vi "Tokenize Json String.vi"(0 "JSON String":string="{\n   \"data\":[\n      {\n         \"message\":{\n            \"content\":{\n               \"type\":\"text/plain\",\n               \"text\":\"Some text asd\"\n            },\n            \"subject\":\"My subject\",\n            \"status\":\"published\",\n            \"replyCount\":4.8,\n            \"likeCount\":0.7\n         }\n      }\n   ]\n}", 11 "Error In":errorcluster) -> (4 "Datatype Tokens":T1[](array[typedef]), 6 "Variable Names":string[](array[string]), 15 "Error Out":errorcluster)   [LabVIEW 2019, in "JsonToCluster.lvlib"]
doc: "This VI converts JSON string into its equivalent tokens as arrays, Clusters and other data types also extracts its label"
uses:
  JsonToCluster.lvlib
  _Controls/Tokens.ctl
  <vilib>/regexp/Match Regular Expression.xnode
panel:
  out "JSON Tokens":string[](array[string])
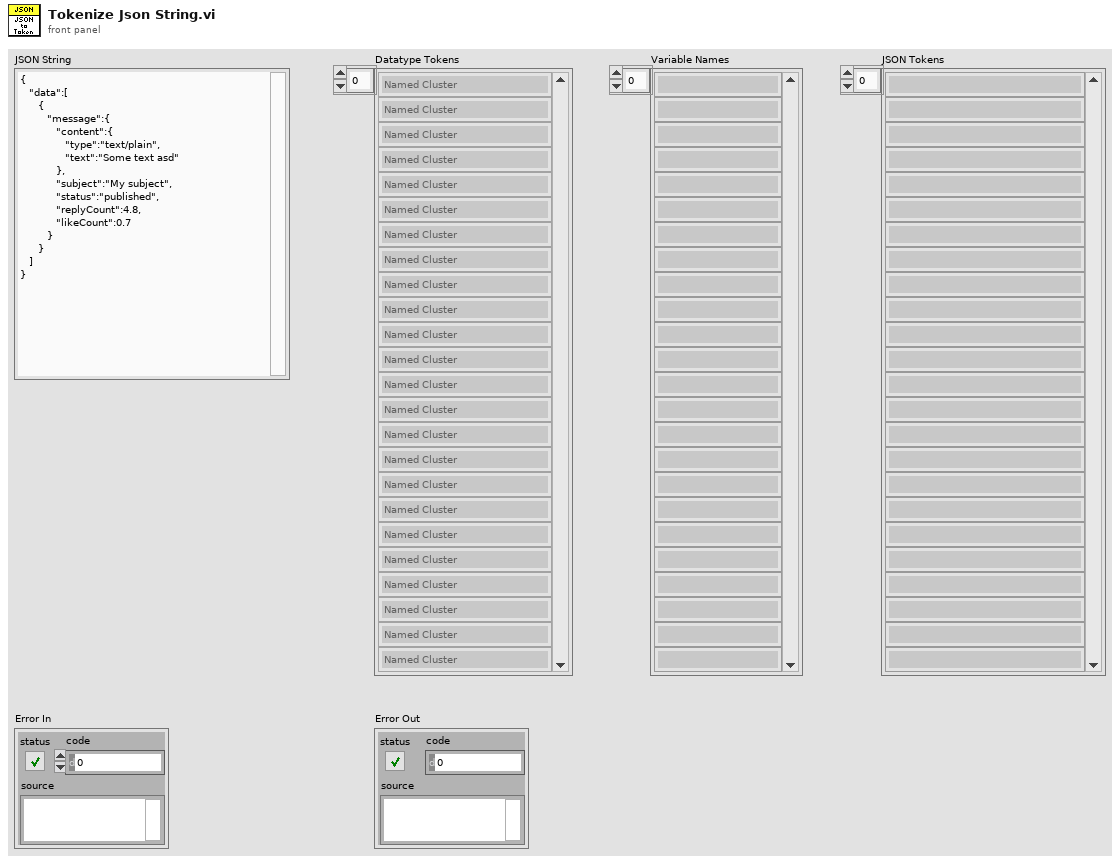
[diagram p1: front panel]
types:
  T1 = typedef "JsonToCluster.lvlib/Tokens.ctl" = enum16{"End", "Boolean", "Named Cluster", "Unnamed Cluster", "Array", "String", "Decimal", "FloatingPoint", "End Array", "End Cluster"}
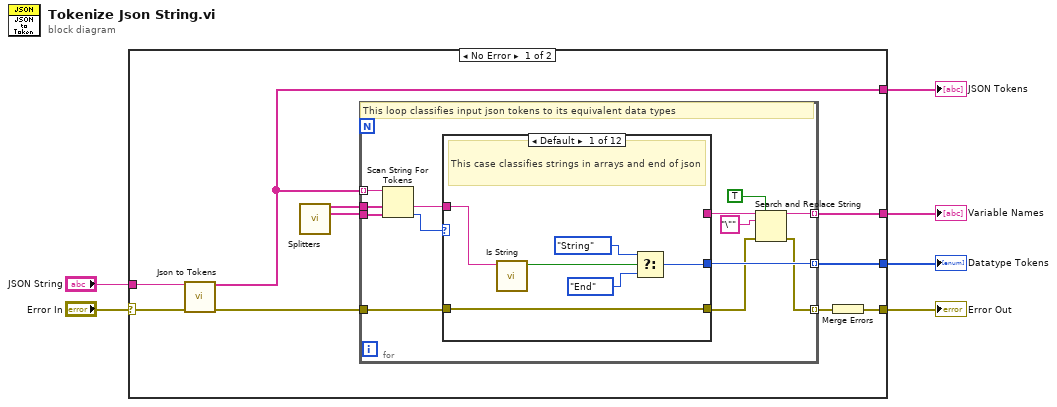
[diagram p0: block diagram]
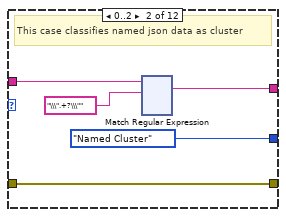
[diagram p2: hidden frame]
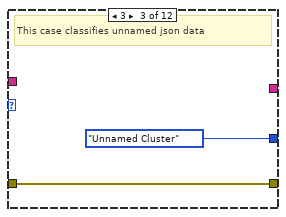
[diagram p3: hidden frame]
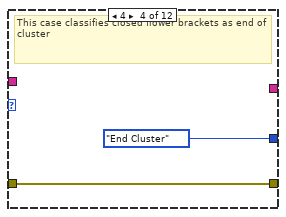
[diagram p4: hidden frame]
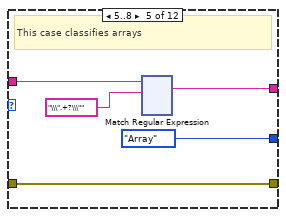
[diagram p5: hidden frame]
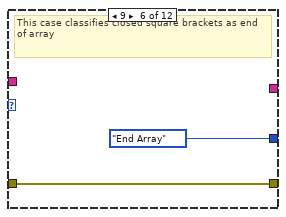
[diagram p6: hidden frame]
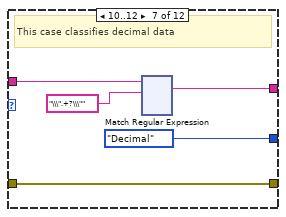
[diagram p7: hidden frame]
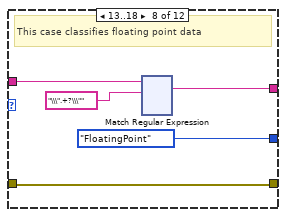
[diagram p8: hidden frame]
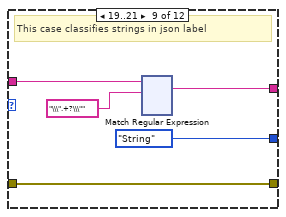
[diagram p9: hidden frame]
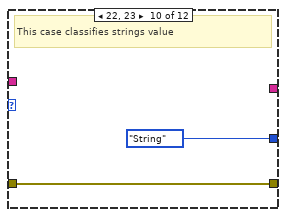
[diagram p10: hidden frame]
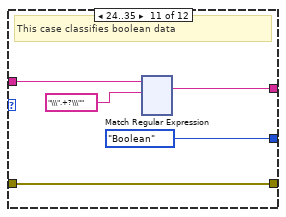
[diagram p11: hidden frame]
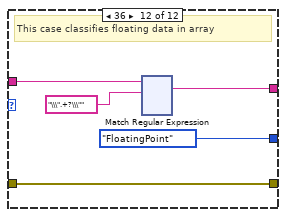
[diagram p12: hidden frame]
diagram:
  n1 = case shown="No Error" "Error In" {
    selector: "Error In" -> [w12 w877]
    tunnel: "JSON String" -> [w16 _]
    tunnel: [w15 _] -> w5
    tunnel: [w14 _] -> w4
    tunnel: [w13 _] -> w3
    tunnel: [w7 w877] -> w1
    frame No Error {
      n2 = call "Json to Tokens.vi"("JSON String"=w16, "Error In"=w12) -> ("JSON Tokens"=w15:string[], "Error Out"=w9:errorcluster)  [unwired: 12 in]
      n3 = call "Splitters.vi"() -> ("Operators"=w11:string[], "Delimiters"=w10:string[])  [unwired: 14 in]
      n4 = for {
        tunnel: w15 -> [w29] mode=indexing
        tunnel: w10 -> [w28]
        tunnel: w11 -> [w27]
        tunnel: [w25] -> w14 mode=indexing
        tunnel: [w22] -> w13 mode=indexing
        tunnel: w9 -> [w19]
        tunnel: [w17] -> w8 mode=indexing
        # "This loop classifies input json tokens to its equivalent data types"
        n5 = Scan String For Tokens(6:w28, 7:w27, 9:w29) -> (0:w26:i32, 1:w24:string)  [unwired: 3 in, 2 out]
        n6 = case shown="Default" w26 {
          tunnel: [w31 Tokens."Named Cluster" Tokens."Unnamed Cluster" Tokens."End Cluster" Tokens."Array" Tokens."End Array" Tokens."Decimal" Tokens."FloatingPoint" Tokens."String" Tokens."String" Tokens."Boolean" Tokens."FloatingPoint"] -> w25
          tunnel: w24 -> [w35 w38 _ _ w161 _ w282 w401 w520 _ w641 w760]
          tunnel: [_ w37 _ _ w160 _ w281 w400 w519 _ w640 w759] -> w23
          tunnel: w19 -> [w30 w36 w155 w157 w159 w278 w280 w399 w518 w637 w639 w758]
          tunnel: [w30 w36 w155 w157 w159 w278 w280 w399 w518 w637 w639 w758] -> w18
          frame Default {
            # "This case classifies strings in arrays and end of json"
            n7 = call "Is String.vi"("Input String"=w35) -> ("Is String?"=w34:bool)  [unwired: 10 in]
            n8 = Select(t=Tokens."String", s=w34, f=Tokens."End") -> (s? t:f=w31:T1)
          }
          frame 0..2 {
            # "This case classifies named json data as cluster"
            n9 = xnode "Match Regular Expression"("input string"=w38, "regular expression"="\\\".+?\\\"") -> ("whole match"=w37:string)  [unwired: 4 in, 4 out]
          }
          frame 3 {
            # "This case classifies unnamed json data"
          }
          frame 4 {
            # "This case classifies closed flower brackets as end of cluster"
          }
          frame 5..8 {
            # "This case classifies arrays"
            n10 = xnode "Match Regular Expression"("input string"=w161, "regular expression"="\\\".+?\\\"") -> ("whole match"=w160:string)  [unwired: 4 in, 4 out]
          }
          frame 9 {
            # "This case classifies closed square brackets as end of array"
          }
          frame 10..12 {
            # "This case classifies decimal data"
            n11 = xnode "Match Regular Expression"("input string"=w282, "regular expression"="\\\".+?\\\"") -> ("whole match"=w281:string)  [unwired: 4 in, 4 out]
          }
          frame 13..18 {
            # "This case classifies floating point data"
            n12 = xnode "Match Regular Expression"("input string"=w401, "regular expression"="\\\".+?\\\"") -> ("whole match"=w400:string)  [unwired: 4 in, 4 out]
          }
          frame 19..21 {
            # "This case classifies strings in json label"
            n13 = xnode "Match Regular Expression"("input string"=w520, "regular expression"="\\\".+?\\\"") -> ("whole match"=w519:string)  [unwired: 4 in, 4 out]
          }
          frame 22, 23 {
            # "This case classifies strings value"
          }
          frame 24..35 {
            # "This case classifies boolean data"
            n14 = xnode "Match Regular Expression"("input string"=w641, "regular expression"="\\\".+?\\\"") -> ("whole match"=w640:string)  [unwired: 4 in, 4 out]
          }
          frame 36 {
            # "This case classifies floating data in array"
            n15 = xnode "Match Regular Expression"("input string"=w760, "regular expression"="\\\".+?\\\"") -> ("whole match"=w759:string)  [unwired: 4 in, 4 out]
          }
        }
        n16 = Search and Replace String(replace all?=TRUE ("replace all? (F)"), input string=w23, search string="\"", error in=w18) -> (result string=w22:string, error out=w17:errorcluster)  [unwired: 4 in, 2 out]
      }
      n17 = Merge Errors(w8) -> (w7:errorcluster)
    }
    frame Error {
    }
  }
  "Datatype Tokens" <- w4
  "Variable Names" <- w3
  "JSON Tokens" <- w5
  "Error Out" <- w1
